vi "Set Force.vi"(8 "error in (no error)":errorcluster, 9 "Force Data":u8[](array[numeric]) format="%.0x", 10 "Force Active":bool, 11 "CIFChannels in":refnum<class "CIFChannels.lvclass">) -> (0 "error out":errorcluster, 3 "CIFChannels out":refnum<class "CIFChannels.lvclass">)   [LabVIEW 2021, in "CIFChannels.lvclass"]
uses:
  CIFChannels.lvclass
  CIFChannels.lvclass/CIFChannels.ctl
  Accessors/Write Tag Forced.vi
  Accessors/Read Direction.vi
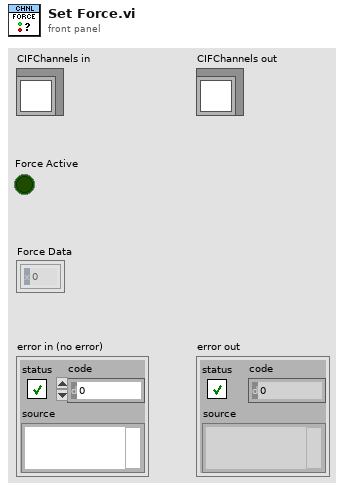
[diagram p1: front panel]
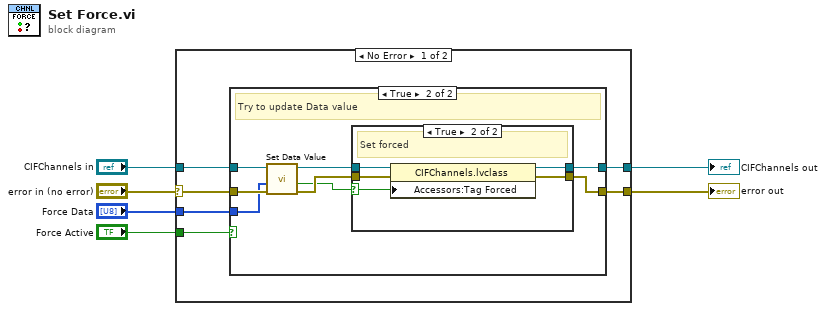
[diagram p0: block diagram]
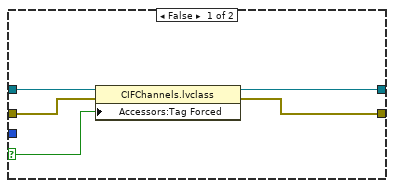
[diagram p2: hidden frame]
diagram:
  n1 = case shown="No Error" "error in (no error)" {
    selector: "error in (no error)" -> [w7 w34]
    tunnel: [w10 w34] -> w5
    tunnel: [w11 w33] -> w1
    tunnel: "CIFChannels in" -> [w8 w33]
    tunnel: "Force Active" -> [w12 _]
    tunnel: "Force Data" -> [w9 _]
    frame No Error {
      n2 = case shown="True" w12 {
        selector: w12 -> [w15 _]
        tunnel: w8 -> [w17 w25]
        tunnel: w7 -> [w16 w24]
        tunnel: [w14 w19] -> w11
        tunnel: [w13 w18] -> w10
        tunnel: w9 -> [_ w23]
        frame False {
          n3 = property class="CIFChannels.lvclass"(reference=w17, error in=w16, "Accessors:Tag Forced"=w15) -> (reference out=w14:refnum<class "CIFChannels.lvclass">, error out=w13:errorcluster)
        }
        frame True {
          # "Try to update Data value"
          n4 = call-dynamic "Set Data Value.vi"("error in (no error)"=w24, "Flat Data"=w23, "CIFChannels in"=w25) -> ("error out"=w21:errorcluster, "Updated"=w20:bool, "CIFChannels out"=w22:refnum<class "CIFChannels.lvclass">)  [unwired: 6 in]
          n5 = case shown="True" w20 {
            selector: w20 -> [_ w30]
            tunnel: w22 -> [w27 w32]
            tunnel: w21 -> [w26 w31]
            tunnel: [w27 w29] -> w19
            tunnel: [w26 w28] -> w18
            frame False {
              # "Update failed"
            }
            frame True {
              # "Set forced"
              n6 = property class="CIFChannels.lvclass"(reference=w32, error in=w31, "Accessors:Tag Forced"=w30) -> (reference out=w29:refnum<class "CIFChannels.lvclass">, error out=w28:errorcluster)
            }
          }
        }
      }
    }
    frame Error {
    }
  }
  "error out" <- w5
  "CIFChannels out" <- w1
